vi "Get_Info_Before-After_Tracks-1.vi"(2 "[IN] After Tracks":T1(array[cluster]), 3 "[IN] Tracks group":i32 min=0 max=399, 4 "[IN] Before Tracks":T1(array[cluster])) -> (0 "[OUT] Maximal Frame\n(finish point all tracks)":i32, 1 "[OUT] Min Start Pos":i32)   [LabVIEW 2013]
doc: "Here the calculation of minimal and maximal indicies of diplacements is performed. This info is valuable for further saving and representation of connected tracks"
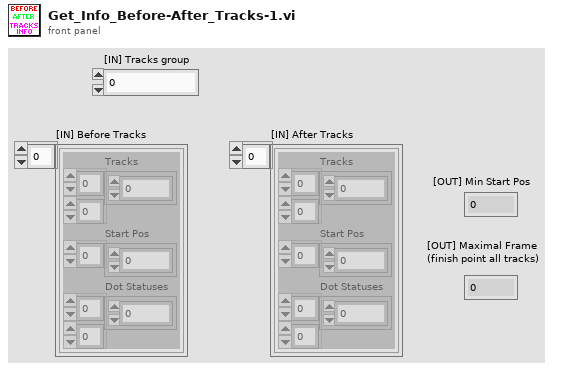
[diagram p1: front panel]
types:
  T1 = cluster{"Tracks":dbl[][], "Start Pos":i32[], "Dot Statuses":i16[][]}[]
  T2 = cluster{"Tracks":dbl[][], "Start Pos":i32[], "Dot Statuses":i16[][]}
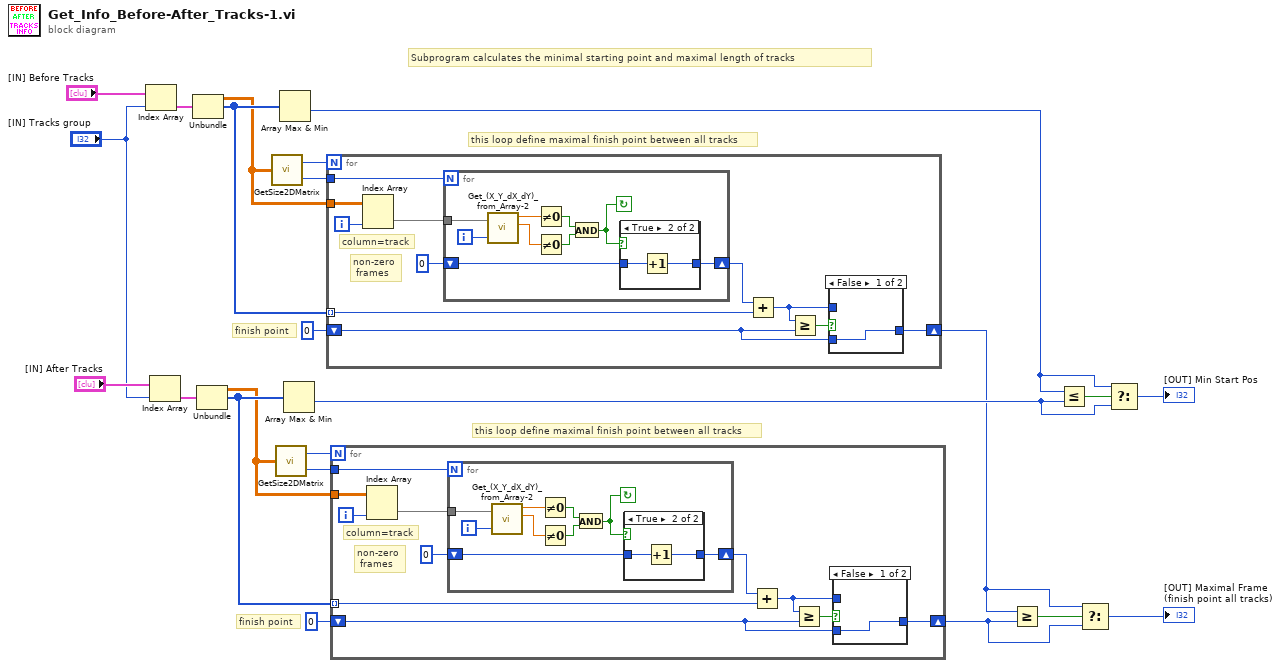
[diagram p0: block diagram]
diagram:
  # "Subprogram calculates the minimal starting point and maximal length of tracks"
  # "finish point"
  # "this loop define maximal finish point between all tracks"
  # "finish point"
  # "this loop define maximal finish point between all tracks"
  n1 = Index Array(array="[IN] Before Tracks", index="[IN] Tracks group") -> (element=w23:T2)
  n2 = Index Array(array="[IN] After Tracks", index="[IN] Tracks group") -> (element=w16:T2)
  n3 = Unbundle(w23) -> ("Tracks"=w18:dbl[][], "Start Pos"=w21:i32[])  [unwired: 1 out]
  n4 = Unbundle(w16) -> ("Tracks"=w12:dbl[][], "Start Pos"=w14:i32[])  [unwired: 1 out]
  n5 = call "GetSize2DMatrix.vi"("Array IN (2D)"=w18) -> ("# Cols"=w22:i32, "# Rows"=w17:i32)
  n6 = call "GetSize2DMatrix.vi"("Array IN (2D)"=w12) -> ("# Cols"=w15:i32, "# Rows"=w11:i32)
  n7 = Array Max & Min(array=w21) -> (min value=w7:i32)  [unwired: 3 out]
  n8 = Array Max & Min(array=w14) -> (min value=w6:i32)  [unwired: 3 out]
  n9 = for {
    N: w22 -> [_]
    tunnel: w18 -> [w34]
    tunnel: w21 -> [w29] mode=indexing
    shift-right: [w26] -> w3
    shift-left: 0 -> [w25]
    tunnel: w17 -> [w24]
    i -> [w33]
    # "non-zero\n frames"
    # "column=track"
    n10 = Index Array(array=w34, index (col)=w33) -> (element=w32:dbl[])  [unwired: 1 in]
    n11 = for {
      N: w24 -> [_]
      tunnel: w32 -> [w40]
      shift-right: [w41] -> w30
      shift-left: 0 -> [w42]
      i -> [w39]
      stop <- w43 continue-if-true
      n12 = call "Get_(X_Y_dX_dY)_from_Array-2.vi"("(X,Y,dX,dY)"=w40, "Index of Displacement"=w39) -> ("X"=w38:dbl, "Y"=w37:dbl)  [unwired: 2 out]
      n13 = Not Equal To 0?(x=w38) -> (x != 0?=w45:bool)
      n14 = Not Equal To 0?(x=w37) -> (x != 0?=w44:bool)
      n15 = And(x=w45, y=w44) -> (x .and. y?=w43:bool)
      n16 = case shown="True" w43 {
        tunnel: w42 -> [w46 w48]
        tunnel: [w46 w47] -> w41
        frame False {
        }
        frame True {
          n17 = Increment(x=w48) -> (x+1=w47:i32)
        }
      }
    }
    n18 = Add(x=w30, y=w29) -> (x+y=w27:i32)
    n19 = Greater Or Equal?(x=w27, y=w25) -> (x >= y?=w28:bool)
    n20 = case shown="False" w28 {
      tunnel: w27 -> [_ w36]
      tunnel: [w35 w36] -> w26
      tunnel: w25 -> [w35 _]
      frame False {
      }
      frame True {
      }
    }
  }
  n21 = for {
    N: w15 -> [_]
    tunnel: w12 -> [w59]
    tunnel: w14 -> [w54] mode=indexing
    shift-right: [w51] -> w2
    shift-left: 0 -> [w50]
    tunnel: w11 -> [w49]
    i -> [w58]
    # "non-zero\n frames"
    # "column=track"
    n22 = Index Array(array=w59, index (col)=w58) -> (element=w57:dbl[])  [unwired: 1 in]
    n23 = for {
      N: w49 -> [_]
      tunnel: w57 -> [w65]
      shift-right: [w66] -> w55
      shift-left: 0 -> [w67]
      i -> [w64]
      stop <- w68 continue-if-true
      n24 = call "Get_(X_Y_dX_dY)_from_Array-2.vi"("(X,Y,dX,dY)"=w65, "Index of Displacement"=w64) -> ("X"=w63:dbl, "Y"=w62:dbl)  [unwired: 2 out]
      n25 = Not Equal To 0?(x=w63) -> (x != 0?=w70:bool)
      n26 = Not Equal To 0?(x=w62) -> (x != 0?=w69:bool)
      n27 = And(x=w70, y=w69) -> (x .and. y?=w68:bool)
      n28 = case shown="True" w68 {
        tunnel: w67 -> [w71 w73]
        tunnel: [w71 w72] -> w66
        frame False {
        }
        frame True {
          n29 = Increment(x=w73) -> (x+1=w72:i32)
        }
      }
    }
    n30 = Add(x=w55, y=w54) -> (x+y=w52:i32)
    n31 = Greater Or Equal?(x=w52, y=w50) -> (x >= y?=w53:bool)
    n32 = case shown="False" w53 {
      tunnel: w52 -> [_ w61]
      tunnel: [w60 w61] -> w51
      tunnel: w50 -> [w60 _]
      frame False {
      }
      frame True {
      }
    }
  }
  n33 = Greater Or Equal?(x=w3, y=w2) -> (x >= y?=w4:bool)
  n34 = Less Or Equal?(x=w7, y=w6) -> (x <= y?=w8:bool)
  n35 = Select(t=w3, s=w4, f=w2) -> (s? t:f=→"[OUT] Maximal Frame\n(finish point all tracks)":i32)
  n36 = Select(t=w7, s=w8, f=w6) -> (s? t:f=→"[OUT] Min Start Pos":i32)
